vi "(SubVI)Scope_Cal Min, Max, Avg.vi"(5 "Num of Register (for Init)":i32, 7 "Init":bool, 8 "error in (no error)":errorcluster caption="에러 입력(에러 없음)", 10 "Count":u16, 11 "Data":i16[][](array[numeric])) -> (0 "error out":errorcluster caption="에러 출력", 3 "Data":string[][](array[string]))   [LabVIEW 2020]
uses:
  <vilib>/Analysis/baseanly.llb/Mean (DBL).vi
  <vilib>/Analysis/NI_AALBase.lvlib
panel:
  # "(SubVI)Scope_Cal Min, Max, Avg.vi By hspark\n\nDescription : Scope 데이터에서 최소, 최대, 평균 값을 계산하여 2D 문자열 배열로 출력하는 VI\n\nInput : \n1. Data : Scope 데이터 입력\n2. Count : 최소, 최대, 평균 값을 계산할 데이터의 수\n3. Init : True 입력 시 초기화\n4. Num of Register (for Init) : 초기화 시 Scope 기능에서 설정한 Register 수 입력\n\nOutput : \n1. Data : 여러열 리스트박스 업데이트를 위해 최근 값 및 계산 결과를 2D 문자열 배열로 출력\n\nLabVIEW Version : 2020 SP1 이상\n\nNote :\n최소, 최대, 평균 값 계산은 Moving Average 방식으로 계산됨.\n따라서 이 VI를 실행할 때 마다 값이 업데이트됨.\n\nUpdate : 2021.10.06"
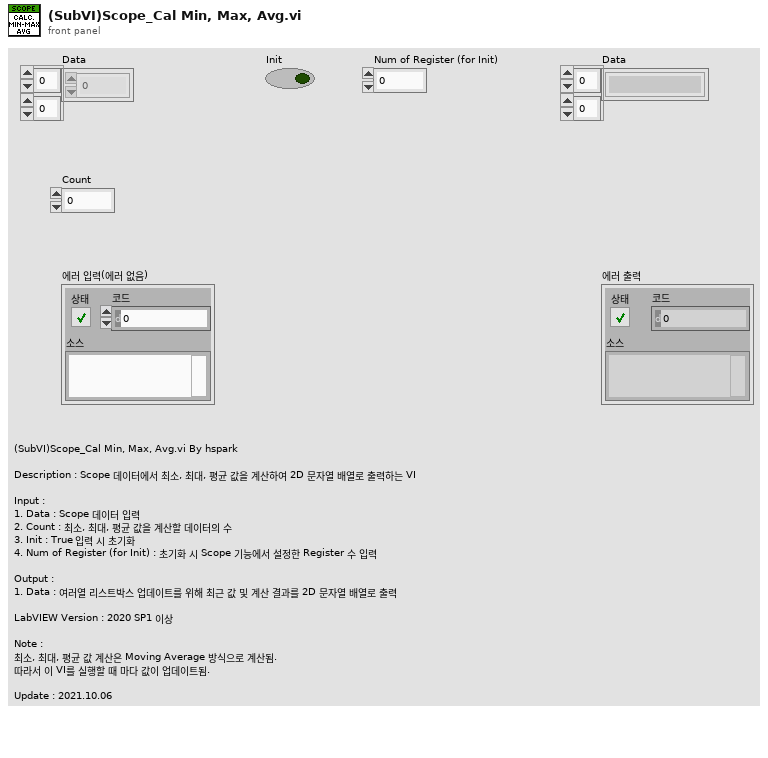
[diagram p1: front panel]
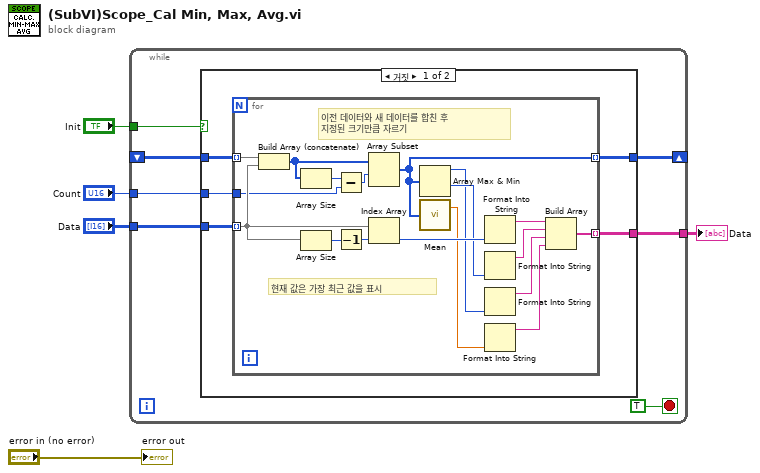
[diagram p0: block diagram]
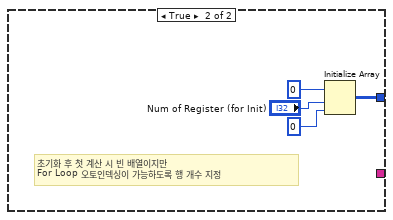
[diagram p2: hidden frame]
diagram:
  n1 = while {
    tunnel: "Data" -> [w12]
    shift-right: [w11] -> _
    shift-left: _ -> [w10]
    tunnel: "Init" -> [w8]
    tunnel: "Count" -> [w7]
    tunnel: [w6] -> w2
    stop <- TRUE stop-if-true
    n2 = case shown="거짓" w8 {
      tunnel: w12 -> [w17 _]
      tunnel: [w15 w36] -> w11
      tunnel: w10 -> [w16 _]
      tunnel: w7 -> [w14 _]
      tunnel: [w13 _] -> w6
      frame False {
        n3 = for {
          tunnel: w17 -> [w33] mode=indexing
          tunnel: w16 -> [w35] mode=indexing
          tunnel: [w34] -> w15 mode=indexing
          tunnel: w14 -> [w27]
          tunnel: [w20] -> w13 mode=indexing
          # "현재 값은 가장 최근 값을 표시"
          # "이전 데이터와 새 데이터를 합친 후\n지정된 크기만큼 자르기"
          n4 = Build Array (concatenate)(w35, w33) -> (w30:i16[])
          n5 = Array Size(array=w30) -> (size(s)=w29:i32)
          n6 = Array Size(array=w33) -> (size(s)=w32:i32)
          n7 = Subtract(x=w29, y=w27) -> (x-y=w28:i32)
          n8 = Decrement(x=w32) -> (x-1=w31:i32)
          n9 = Array Subset(array=w30, index=w28) -> (w34:i16[])  [unwired: 1 in]
          n10 = Index Array(array=w33, index=w31) -> (element=w26:i16)
          n11 = Array Max & Min(array=w34) -> (max value=w18:i16, min value=w19:i16)  [unwired: 2 out]
          n12 = call-poly <vilib>:"Mean.vi"("X"=w34) -> ("mean"=w25:dbl)  [unwired: 1 out]
          n13 = Format Into String(w26) -> (resulting string=w24:string)  [unwired: 3 in, 1 out]
          n14 = Format Into String(w19) -> (resulting string=w23:string)  [unwired: 3 in, 1 out]
          n15 = Format Into String(w18) -> (resulting string=w22:string)  [unwired: 3 in, 1 out]
          n16 = Format Into String(w25) -> (resulting string=w21:string)  [unwired: 3 in, 1 out]
          n17 = Build Array(w24, w23, w22, w21) -> (w20:string[])
        }
      }
      frame True {
        # "초기화 후 첫 계산 시 빈 배열이지만\nFor Loop 오토인덱싱이 가능하도록 행 개수 지정"
        n18 = Initialize Array(i16 0, "Num of Register (for Init)", 0 ("차원 크기")) -> (w36:i16[][])
      }
    }
  }
  "Data" <- w2
  "error out" <- "error in (no error)"
